vi "Global 2.vi"() -> ()   [LabVIEW 2011]
uses:
  <vilib>/Simulation/Param Hierarchy/Typedefs/SIMPH System.ctl
  <vilib>/Simulation/Param Hierarchy/Typedefs/SIMPH Block.ctl
  <vilib>/Simulation/Param Hierarchy/Typedefs/SIMPH Param Source.ctl
panel:
  in  "SIMPH Param Buffer":T1={"Sine Signal"={"amplitude"=1.0, "offset"=0.0, "frequency"=0.5, "phase"=0.0, "output"=0.0}, "Simulation Time Waveform"={"Value"=0.0, "Waveform Chart"={"t0"=timestamp(9343.2 s since 1904-01-01), "dt"=1.0, "Y"=[0.2633720690985406]}}}
  in  "SIMPH Block Array":T2=[{"Type"=0, "Child Block Count"=2, "Parameters"=[], "Name"="NILVSim_Top_Level_Subsystem"}, {"Type"=28, "Child Block Count"=0, "Parameters"=[{"Name"="amplitude", "Source"=enum."Param (Config)"}, {"Name"="offset", "Source"=enum."Param (Config)"}, {"Name"="frequency", "Source"=enum."Param (Wired)"}, {"Name"="phase", "Source"=enum."Param (Config)"}, {"Name"="output", "Source"=enum."Output"}], "Name"="Sine Signal"}, {"Type"=48, "Child Block Count"=0, "Parameters"=[{"Name"="Value", "Source"=enum."Input"}, {"Name"="Waveform Chart", "Source"=enum."Output"}], "Name"="Simulation Time Waveform"}]
  out "SIMPH Params Dirty":bool
  out "SIMPH Params Changed":bool
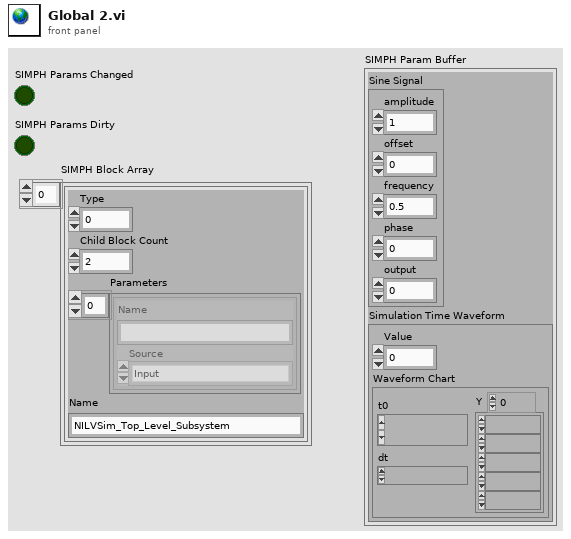
[diagram p1: front panel]
types:
  T1 = cluster{"Sine Signal":cluster{"amplitude":dbl, "offset":dbl, "frequency":dbl, "phase":dbl, "output":dbl}, "Simulation Time Waveform":cluster{"Value":dbl, "Waveform Chart":waveform(dbl)}}
  T2 = typedef "SIMPH System.ctl" = T3[]
  T3 = typedef "SIMPH Block.ctl" = cluster{"Type":u32, "Child Block Count":u32, "Parameters":cluster{"Name":string, "Source":T4}[], "Name":string}
  T4 = typedef "SIMPH Param Source.ctl" = enum16{"Input", "Output", "Param (Wired)", "Param (Unwired)", "Param (Config)"}
diagram:
